vi "Read Function Parameters.vi"(0 "signal configuration":refnum<class "SV Function.lvclass">, 11 "error in (no error)":errorcluster) -> (3 "function type":u16(ring) items=["Sine", "Triangle", "Square", "Sawtooth"], 4 "signal configuration":refnum<class "SV Function.lvclass">, 6 "frequency_Hz":dbl=1000.0, 8 "amplitude":dbl=1.0, 10 "initial_phase_deg":dbl, 15 "error out":errorcluster)   [LabVIEW 2017, in "SV Function.lvclass"]
uses:
  <vilib>/addons/_NISVFA/_Generation/Signal Generation/SV Function/SV Function.lvclass
  <vilib>/addons/_NISVFA/_Generation/Signal Generation/SV Function/SV Function.lvclass/SV Function.ctl
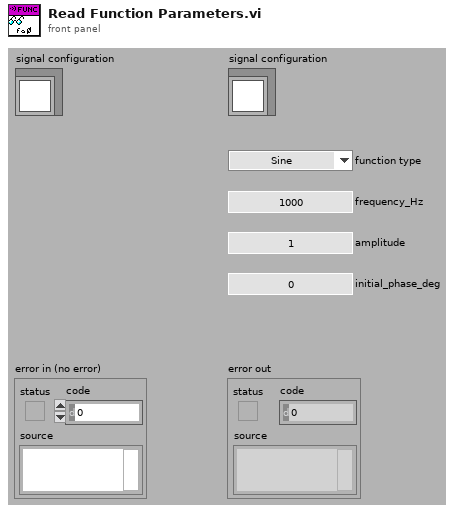
[diagram p1: front panel]
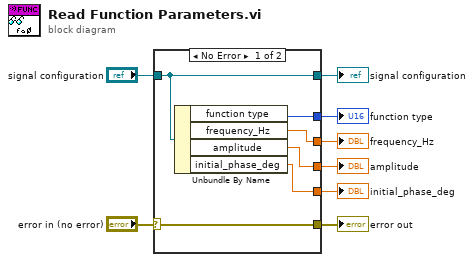
[diagram p0: block diagram]
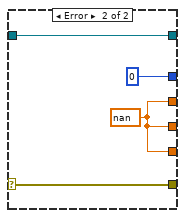
[diagram p2: hidden frame]
diagram:
  n1 = case shown="No Error" "error in (no error)" {
    selector: "error in (no error)" -> [w14 w17]
    tunnel: [w14 w17] -> w7
    tunnel: [w13 w18] -> w5
    tunnel: "signal configuration" -> [w13 w18]
    tunnel: [w12 w15] -> w4
    tunnel: [w11 u16 0 ("function type")] -> w3
    tunnel: [w10 w15] -> w2
    tunnel: [w9 w15] -> w1
    frame No Error {
      n2 = Unbundle By Name(w13) -> ("function type"=w11:u16, "frequency_Hz"=w10:dbl, "amplitude"=w9:dbl, "initial_phase_deg"=w12:dbl)
    }
    frame Error {
      w15 = nan ("frequency_Hz")
    }
  }
  "error out" <- w7
  "signal configuration" <- w5
  "initial_phase_deg" <- w4
  "function type" <- w3
  "amplitude" <- w1
  "frequency_Hz" <- w2
